vi "Generate new values for S and P.vi"() -> ()   [LabVIEW 2022 SP3, in "Registration.lvclass"]
uses:
  Registration.lvclass
panel:
  out "Generated P Array U8x72":u8[](array[numeric]) format="%.0x"
  out "Generated S Box U32x4x256":u32[][](array[numeric]) format="%.0x"
  # "Save these values.\nThe P and S values must be the same as when decypting\nthe message.  If not you will not be able to recover your\ndata."
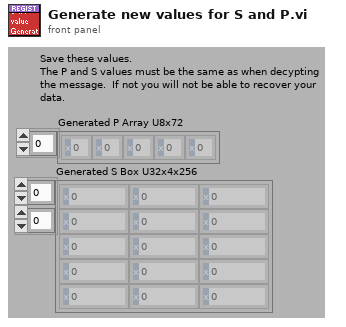
[diagram p1: front panel]
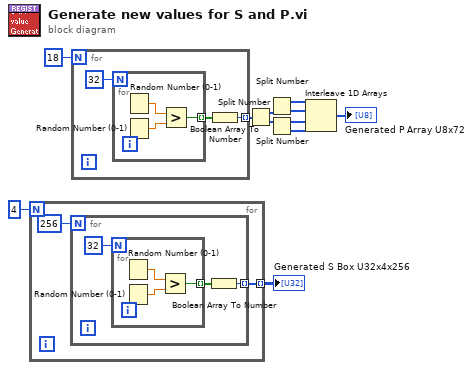
[diagram p0: block diagram]
diagram:
  n1 = for {
    N: 4 -> [_]
    tunnel: [w12] -> w2 mode=indexing
    n2 = for {
      N: 256 -> [_]
      tunnel: [w14] -> w12 mode=indexing
      n3 = for {
        N: 32 -> [_]
        tunnel: [w17] -> w16 mode=indexing
        n4 = Random Number (0-1)() -> (number: 0 to 1=w19:dbl)
        n5 = Random Number (0-1)() -> (number: 0 to 1=w18:dbl)
        n6 = Greater?(x=w19, y=w18) -> (0:w17:bool)
      }
      n7 = Boolean Array To Number(Boolean array=w16) -> (number=w14:u32)
    }
  }
  "Generated S Box U32x4x256" <- w2
  n8 = for {
    N: 18 -> [_]
    tunnel: [w20] -> w11 mode=indexing
    n9 = for {
      N: 32 -> [_]
      tunnel: [w23] -> w22 mode=indexing
      n10 = Random Number (0-1)() -> (number: 0 to 1=w25:dbl)
      n11 = Random Number (0-1)() -> (number: 0 to 1=w24:dbl)
      n12 = Greater?(x=w25, y=w24) -> (0:w23:bool)
    }
    n13 = Boolean Array To Number(Boolean array=w22) -> (number=w20:u32)
  }
  n14 = Split Number(x=w11) -> (hi(x)=w10:u16[], lo(x)=w9:u16[])
  n15 = Split Number(x=w10) -> (hi(x)=w8:u8[], lo(x)=w7:u8[])
  n16 = Split Number(x=w9) -> (hi(x)=w6:u8[], lo(x)=w5:u8[])
  n17 = Interleave 1D Arrays(w8, w7, w6, w5) -> (→"Generated P Array U8x72":u8[])
